vi "Read Controls.vi"(8 "error in (no error)":errorcluster, 11 "VIEW in":refnum<class "VIEW.lvclass">) -> (0 "error out":errorcluster, 2 "Controls":T1(array[cluster]), 3 "VIEW out":refnum<class "VIEW.lvclass">)   [LabVIEW 2013, in "VIEW.lvclass"]
uses:
  VIEW.lvclass
  VIEW.lvclass/VIEW.ctl
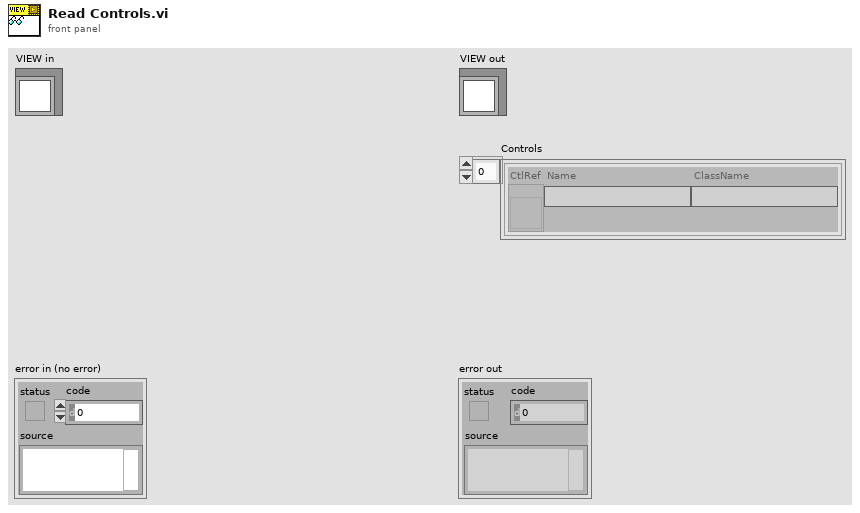
[diagram p1: front panel]
types:
  T1 = cluster{"CtlRef":refnum<vi>, "Name":string, "ClassName":string}[]
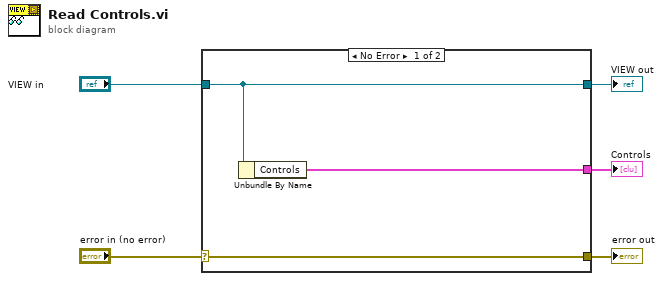
[diagram p0: block diagram]
diagram:
  n1 = case shown="No Error" "error in (no error)" {
    selector: "error in (no error)" -> [w8 w9]
    tunnel: [w8 w9] -> w4
    tunnel: [w7 w10] -> w2
    tunnel: "VIEW in" -> [w7 w10]
    tunnel: [w6 _] -> w1
    frame No Error {
      n2 = Unbundle By Name(w7) -> ("Controls"=w6:T1)
    }
    frame Error {
    }
  }
  "error out" <- w4
  "VIEW out" <- w2
  "Controls" <- w1
